vi "Stop Core.vi"(10 "final error code":i32, 11 "Module in":refnum<class "Module.lvclass">) -> (3 "Module out":refnum<class "Module.lvclass">)   [LabVIEW 2025, in "Module.lvlib" / "Module.lvclass"]
doc: "<p>(<strong>Filename</strong>: <span class=\"dnl\">Actor Framework.lvlib:Actor.lvclass:Stop Core.vi</span>)</p>\n<p>Defines what the actor does before it stops. Use the <strong>final error code</strong> input to determine whether the actor shut down in response to an error.</p>\n<p>By default, this method passes the Stop message along to all <a href=\"nihelplauncher://docs/csh?context=lvcore_lvcomm_af_launch_nested_actor\">auto-stop nested actors</a>. A descendant class may override this method to define additional behavior, such as shutting down any processes the actor initiated in its override of the <a href=\"nihelplauncher://docs/csh?context=lvcore_lvcomm_af_actor_core\">Actor Core</a> method.</p>"
uses:
  Module.lvclass
  <vilib>/ActorFramework/Actor/Actor.lvclass
  Module.lvclass/Module.ctl
  Msg.ctl
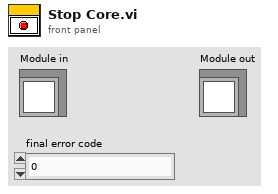
[diagram p1: front panel]
types:
  T1 = typedef "Msg.ctl" = string
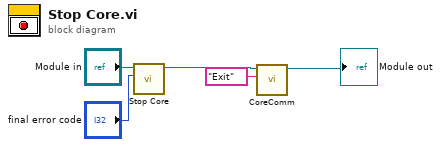
[diagram p0: block diagram]
diagram:
  n1 = call-parent "Stop Core.vi"("final error code"="final error code", "Actor in"="Module in") -> ("Actor out"=w3:refnum<class "Module.lvclass">)  [unwired: 9 in]
  n2 = call-dynamic "CoreComm.vi"("Msg"=T1 "Exit", "Module in"=w3) -> ("Module out"=→"Module out":refnum<class "Module.lvclass">)  [unwired: 8 in, 1 out]
